vi "Cmd to Byte Array (Int).vi"(9 "Parameter":u32, 10 "Commands":T1, 11 "Motor index":u8) -> (2 "Byte string":string)   [LabVIEW 2014, in "Motor manager.lvlib"]
uses:
  Motor manager.lvlib
  Typedef/Commands.ctl
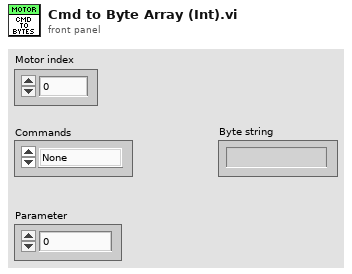
[diagram p1: front panel]
types:
  T1 = typedef "Motor manager.lvlib/Commands.ctl" = enum16{"None", "Set motor", "Set distance", "Set speed", "Set Move Type", "Set IM Idle Time", "Set N cycles", "Start", "Stop", "Stop and Release", "Set Home", "Find Home", "Move Forward", "Move Backward"}
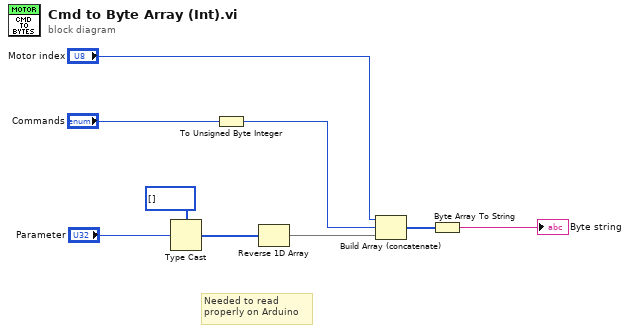
[diagram p0: block diagram]
diagram:
  # "Needed to read \nproperly on Arduino"
  n1 = Type Cast(type=u8[] [], x="Parameter") -> (*(type *) &x=w3:u8[])
  n2 = To Unsigned Byte Integer(number="Commands") -> (unsigned 8bit integer=w8:u8)
  n3 = Reverse 1D Array(array=w3) -> (reversed array=w2:u8[])
  n4 = Build Array (concatenate)("Motor index", w8, w2) -> (w6:u8[])
  n5 = Byte Array To String(unsigned byte array=w6) -> (string=→"Byte string":string)
